vi "UPgetData.vi"() -> ()   [LabVIEW 2020]
panel:
  in  "stop":bool
  in  "Server Closed 2":string="The server VI closed the connection."
  out "data out":string
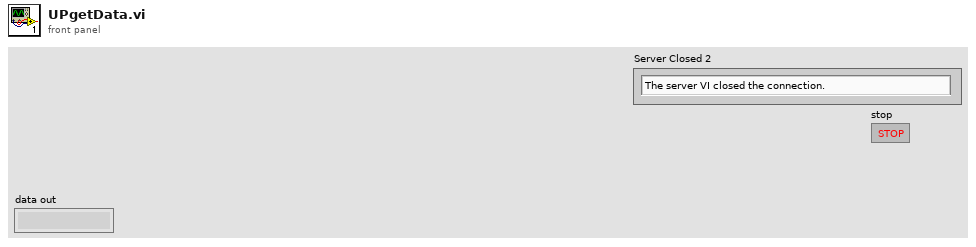
[diagram p1: front panel]
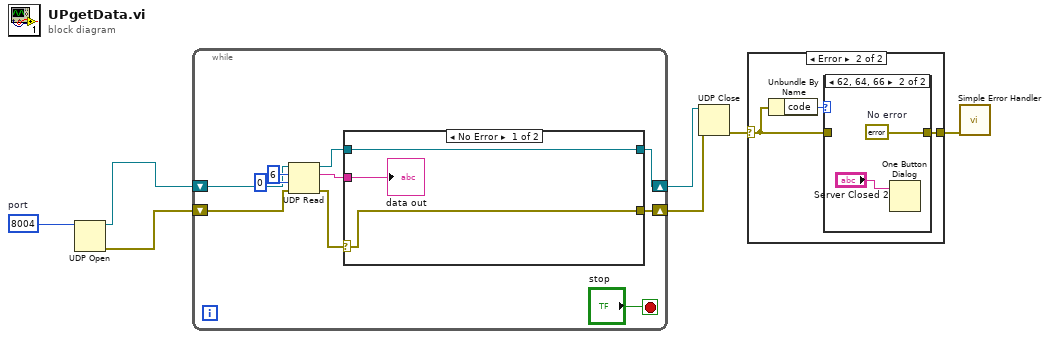
[diagram p0: block diagram]
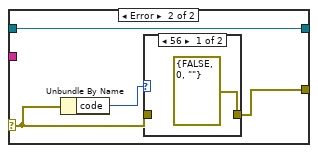
[diagram p2: hidden frame]
diagram:
  w7 = u16 8004  # port
  n1 = UDP Open(11:w7) -> (port=w1:refnum<k16>, 0:w2:errorcluster)  [unwired: 4 in, 1 out]
  n2 = while {
    shift-right: [w11] -> w3
    shift-left: w2 -> [w10]
    shift-right: [w12] -> w4
    shift-left: w1 -> [w9]
    stop <- "stop" stop-if-true
    n3 = UDP Read(connection ID=w9, max size (548)=6, timeout ms (25000)=0, 8:w10) -> (data out=w17:string, error out=w14:errorcluster, 3:w13:refnum<k16>)  [unwired: 2 out]
    n4 = case shown="No Error" w14 {
      selector: w14 -> [w18 w22]
      tunnel: w17 -> [w20 _]
      tunnel: [w19 w23] -> w12
      tunnel: w13 -> [w19 w23]
      tunnel: [w18 w21] -> w11
      frame No Error {
        "data out" <- w20
      }
      frame Error {
        n5 = Unbundle By Name(w22) -> ("code"=w24:i32)
        n6 = case shown="56" w24 {
          tunnel: w22 -> [_ w26]
          tunnel: [errorcluster {FALSE, 0, ""} w26] -> w21
          frame 56 {
          }
          frame Default {
          }
        }
      }
    }
  }
  n7 = UDP Close(connection ID=w4, 8:w3) -> (error out=w6:errorcluster)  [unwired: 1 out]
  n8 = case shown="Error" w6 {
    selector: w6 -> [w27 w29]
    tunnel: [w27 w28] -> w5
    frame No Error {
    }
    frame Error {
      n9 = Unbundle By Name(w29) -> ("code"=w30:i32)
      n10 = case shown="62, 64, 66" w30 {
        tunnel: w29 -> [w31 _]
        tunnel: [w31 w33] -> w28
        frame Default {
        }
        frame 62, 64, 66 {
          w33 = errorcluster {"status"=FALSE, "code"=0, "source"=""}  # No error
          n11 = One Button Dialog(message="Server Closed 2") -> ()  [unwired: 1 in, 1 out]
        }
      }
    }
  }
  n12 = call <vilib>:"Simple Error Handler.vi"("error in (no error)"=w5) -> ()  [unwired: 4 in, 5 out]
